vi "Measurement Controller API Example.vi"() -> ()   [LabVIEW 2016]
uses:
  MAL-Framework/user.lib/Common Components/Results/Results.lvclass
  Controller API.lvclass
panel:
  out "Measurement Results 3":refnum<class "Results.lvclass">
  out "Measurement Results 2":refnum<class "Results.lvclass">
  out "Measurement Results":refnum<class "Results.lvclass">
  out "error out":errorcluster
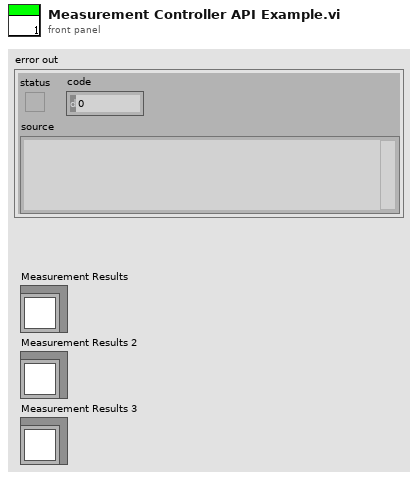
[diagram p1: front panel]
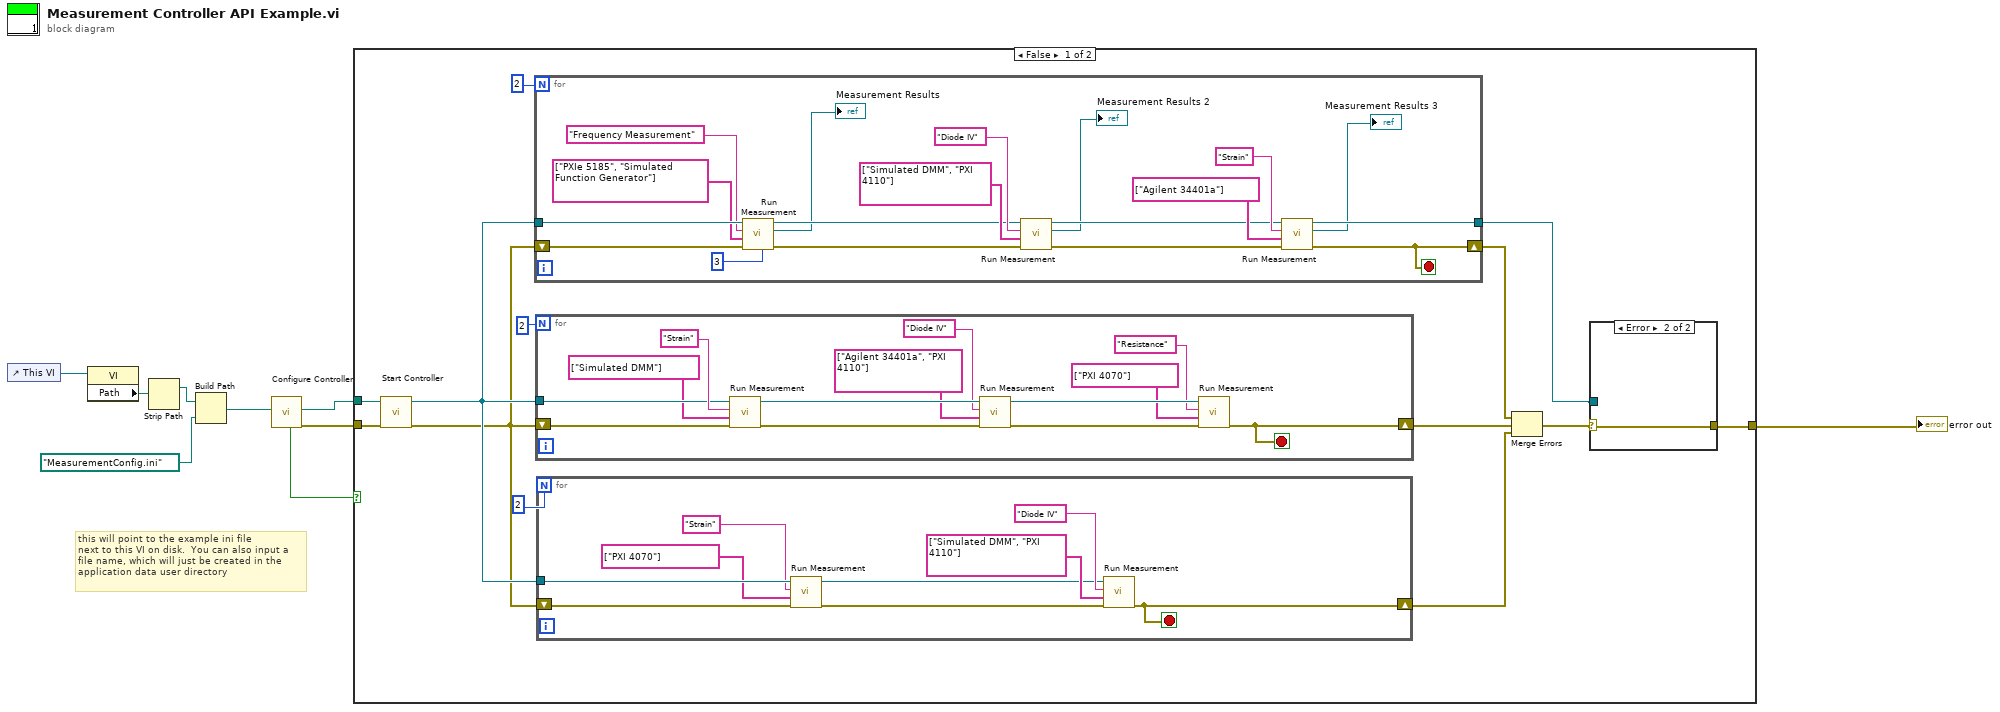
[diagram p0: block diagram]
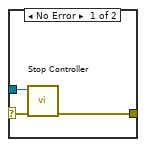
[diagram p2: hidden frame]
diagram:
  # "this will point to the example ini file\nnext to this VI on disk.  You can also input a\nfile name, which will just be created in the \napplication data user directory"
  n1 = control-ref of="This VI"() -> (w9:refnum<vi>)
  n2 = property class="VI"(reference=w9) -> ("Path"=w8:path)  [unwired: 1 in, 2 out]
  n3 = Strip Path(path=w8) -> (stripped path=w7:path)  [unwired: 1 out]
  n4 = Build Path(base path=w7, name or relative path=path "MeasurementConfig.ini" ("Config File Path")) -> (appended path=w5:path)
  n5 = call "Configure Controller.vi"("Config File Path"=w5) -> ("error IO"=w3:errorcluster, "Absolute Path"=w4:path, "Canceled?"=w2:bool)  [unwired: 8 in]
  n6 = case shown="False" w2 {
    tunnel: w4 -> [w14 _]
    tunnel: w3 -> [w13 w67]
    tunnel: [w10 w67] -> w1
    frame False {
      n7 = call "Start Controller.vi"("error in (no error)"=w13, "Config File Path"=w14) -> ("error out"=w15:errorcluster, "Controller Queue"=w22:refnum<class "Message Enqueuer.lvclass">)  [unwired: 7 in, 1 out]
      n8 = for {
        N: 2 -> [_]
        tunnel: w22 -> [w40]
        tunnel: [w39] -> w12
        shift-right: [w34] -> w21
        shift-left: w15 -> [w33]
        stop <- w34 stop-if-true
        n9 = call "Run Measurement.vi"("Iterations"=3, "error in (no error)"=w33, "Device Names"=string[] ["PXIe 5185", "Simulated Function Generator"], "Measurement Name"="Frequency Measurement", "Self Enqueuer In"=w40) -> ("error out"=w37:errorcluster, "Measurement Results"=→"Measurement Results":refnum<class "Results.lvclass">, "Self Enqueuer Out"=w38:refnum<class "Message Enqueuer.lvclass">)  [unwired: 4 in]
        n10 = call "Run Measurement.vi"("error in (no error)"=w37, "Device Names"=string[] ["Simulated DMM", "PXI 4110"], "Measurement Name"="Diode IV", "Self Enqueuer In"=w38) -> ("error out"=w35:errorcluster, "Measurement Results"=→"Measurement Results 2":refnum<class "Results.lvclass">, "Self Enqueuer Out"=w36:refnum<class "Message Enqueuer.lvclass">)  [unwired: 5 in]
        n11 = call "Run Measurement.vi"("error in (no error)"=w35, "Device Names"=string[] ["Agilent 34401a"], "Measurement Name"="Strain", "Self Enqueuer In"=w36) -> ("error out"=w34:errorcluster, "Measurement Results"=→"Measurement Results 3":refnum<class "Results.lvclass">, "Self Enqueuer Out"=w39:refnum<class "Message Enqueuer.lvclass">)  [unwired: 5 in]
      }
      n12 = for {
        N: 2 -> [_]
        tunnel: w22 -> [w65]
        shift-right: [w57] -> w20
        shift-left: w15 -> [w54]
        stop <- w57 stop-if-true
        n13 = call "Run Measurement.vi"("error in (no error)"=w54, "Device Names"=string[] ["Simulated DMM"], "Measurement Name"="Strain", "Self Enqueuer In"=w65) -> ("error out"=w62:errorcluster, "Self Enqueuer Out"=w63:refnum<class "Message Enqueuer.lvclass">)  [unwired: 5 in, 1 out]
        n14 = call "Run Measurement.vi"("error in (no error)"=w62, "Device Names"=string[] ["Agilent 34401a", "PXI 4110"], "Measurement Name"="Diode IV", "Self Enqueuer In"=w63) -> ("error out"=w58:errorcluster, "Self Enqueuer Out"=w59:refnum<class "Message Enqueuer.lvclass">)  [unwired: 5 in, 1 out]
        n15 = call "Run Measurement.vi"("error in (no error)"=w58, "Device Names"=string[] ["PXI 4070"], "Measurement Name"="Resistance", "Self Enqueuer In"=w59) -> ("error out"=w57:errorcluster)  [unwired: 5 in, 2 out]
      }
      n16 = for {
        N: 2 -> [_]
        tunnel: w22 -> [w53]
        shift-right: [w46] -> w19
        shift-left: w15 -> [w45]
        stop <- w46 stop-if-true
        n17 = call "Run Measurement.vi"("error in (no error)"=w45, "Device Names"=string[] ["PXI 4070"], "Measurement Name"="Strain", "Self Enqueuer In"=w53) -> ("error out"=w49:errorcluster, "Self Enqueuer Out"=w48:refnum<class "Message Enqueuer.lvclass">)  [unwired: 5 in, 1 out]
        n18 = call "Run Measurement.vi"("error in (no error)"=w49, "Device Names"=string[] ["Simulated DMM", "PXI 4110"], "Measurement Name"="Diode IV", "Self Enqueuer In"=w48) -> ("error out"=w46:errorcluster)  [unwired: 5 in, 2 out]
      }
      n19 = Merge Errors(w21, w20, w19) -> (w11:errorcluster)
      n20 = case shown="Error" w11 {
        selector: w11 -> [w23 w26]
        tunnel: w12 -> [w25 _]
        tunnel: [w24 w26] -> w10
        frame No Error {
          n21 = call "Stop Controller.vi"("error in (no error)"=w23, "TestStand Controller Queue"=w25) -> ("error out"=w24:errorcluster)  [unwired: 9 in]
        }
        frame Error {
        }
      }
    }
    frame True {
    }
  }
  "error out" <- w1
